vi "Read Core.vi"(8 "error in (no error)":errorcluster, 11 "Display State In in":T1) -> (0 "error out":errorcluster, 2 "Webview2 Core":refnum<k24>, 3 "Display State In in 2":T1)   [LabVIEW 2020, in "WebView2 Control.xctl"]
uses:
  WebView2 Control.xctl
  E:/Labview/LV 2020/Libs/WebView2/LV-WebView2/Source/Libs/Microsoft.Web.WebView2.Core.dll
  Libs/Microsoft.Web.WebView2.Core.dll
  State.ctl
  Events.ctl
  Navigation Event Data.ctl
  Source Changed Event Data.ctl
  Navigation Start Event Data.ctl
  Paths.ctl
  Core Env Options.ctl
  Res.ctl
  E:/Labview/LV 2020/Libs/WebView2/LV-WebView2/Source/Libs/Microsoft.Web.WebView2.WinForms.dll
  Libs/Microsoft.Web.WebView2.WinForms.dll
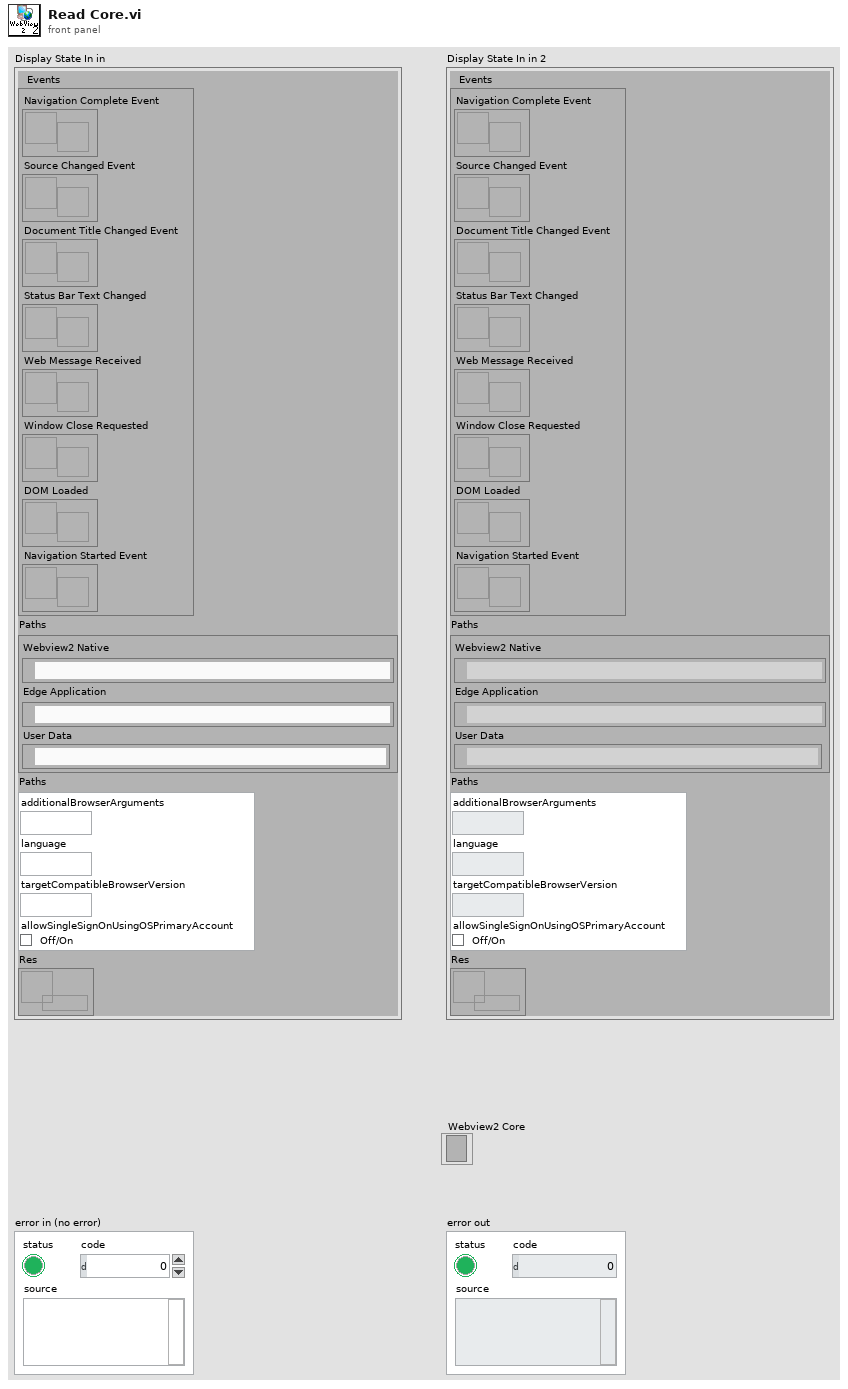
[diagram p1: front panel]
types:
  T1 = typedef "WebView2 Control.xctl/State.ctl" = cluster{"Events":T2, "Paths":T3, "Environment Options":T4, "Res":refnum<data-value>}
  T2 = typedef "WebView2 Control.xctl/Events.ctl" = cluster{"Navigation Complete Event":refnum<user-event>, "Source Changed Event":refnum<user-event>, "Document Title Changed Event":refnum<user-event>, "Status Bar Text Changed":refnum<user-event>, "Web Message Received":refnum<user-event>, "Window Close Requested":refnum<user-event>, "DOM Loaded":refnum<user-event>, "Navigation Started Event":refnum<user-event>}
  T3 = typedef "WebView2 Control.xctl/Paths.ctl" = cluster{"Webview2 Native":path, "Edge Application":path, "User Data":path}
  T4 = typedef "WebView2 Control.xctl/Core Env Options.ctl" = cluster{"additionalBrowserArguments":string, "language":string, "targetCompatibleBrowserVersion":string, "allowSingleSignOnUsingOSPrimaryAccount":bool}
  T5 = typedef "WebView2 Control.xctl/Res.ctl" = cluster{"WebView2":refnum<k24>, "Webview2 Core":refnum<k24>, "event callback":refnum<k27>, "Callbacks":refnum<vi>[]}
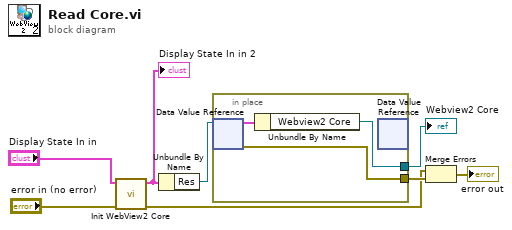
[diagram p0: block diagram]
diagram:
  n1 = call "Init WebView2 Core.vi"("error in (no error)"="error in (no error)", "Display State In"="Display State In in") -> ("error out"=w1:errorcluster, "Display State In 2"=w3:T1)  [unwired: 8 in]
  "Display State In in 2" <- w3
  n2 = Unbundle By Name(w3) -> ("Res"=w5:refnum<data-value>)
  n3 = in-place {
    in-place-border: [w10] -> w6
    in-place-border: [w9] -> w8
    n4 = in-place-dvr #1(w5) -> (w11:T5, w9:errorcluster)
    n5 = Unbundle By Name(w11) -> ("Webview2 Core"=w10:refnum<k24>)
    n6 = in-place-dvr #1() -> ()  [unwired: 1 in, 2 out]
  }
  "Webview2 Core" <- w6
  n7 = Merge Errors(w1, w8) -> (→"error out":errorcluster)
